vi "niRFUtil MT UTIL Calcuate PN Bits Galois.vi"(4 "primitive polynomial coeffs (without MSB)":u32, 6 "Reset? (T)":bool=TRUE, 9 "seed in (0xD6BF7DF2)":T4=3602873842 format="%.0x", 10 "PN Sequence Order (9)":T2=9, 11 "Total Bits":i32) -> (1 "seed out":T4 format="%.0x", 3 "Output Bit Stream":T3 min=0)   [LabVIEW 2015, in "niRFUtil.lvlib"]
doc: "This VI generates a pseudo-random bit stream. The length of the random sequence (i.e., the number of bits that are produced before the pattern repeats itself) is user-defined."
uses:
  niRFUtil.lvlib
  Includes/niRFUtil INC PN Seed.ctl
  Includes/niRFUtil INC Bit Array.ctl
  Includes/niRFUtil INC PN Order.ctl
panel:
  in  "Case Constant\n(See Context Help)":T1(ring)=enum."Shift Primative Seeds"
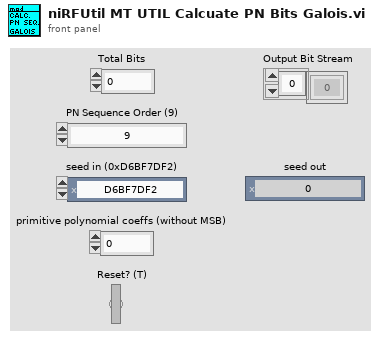
[diagram p1: front panel]
types:
  T1 = enum16{"Ver 2 Algorithm", "Shift Primative Seeds"}
  T2 = typedef "niRFUtil.lvlib/niRFUtil INC PN Order.ctl" = i32
  T3 = typedef "niRFUtil.lvlib/niRFUtil INC Bit Array.ctl" = i8[]
  T4 = typedef "niRFUtil.lvlib/niRFUtil INC PN Seed.ctl" = u32
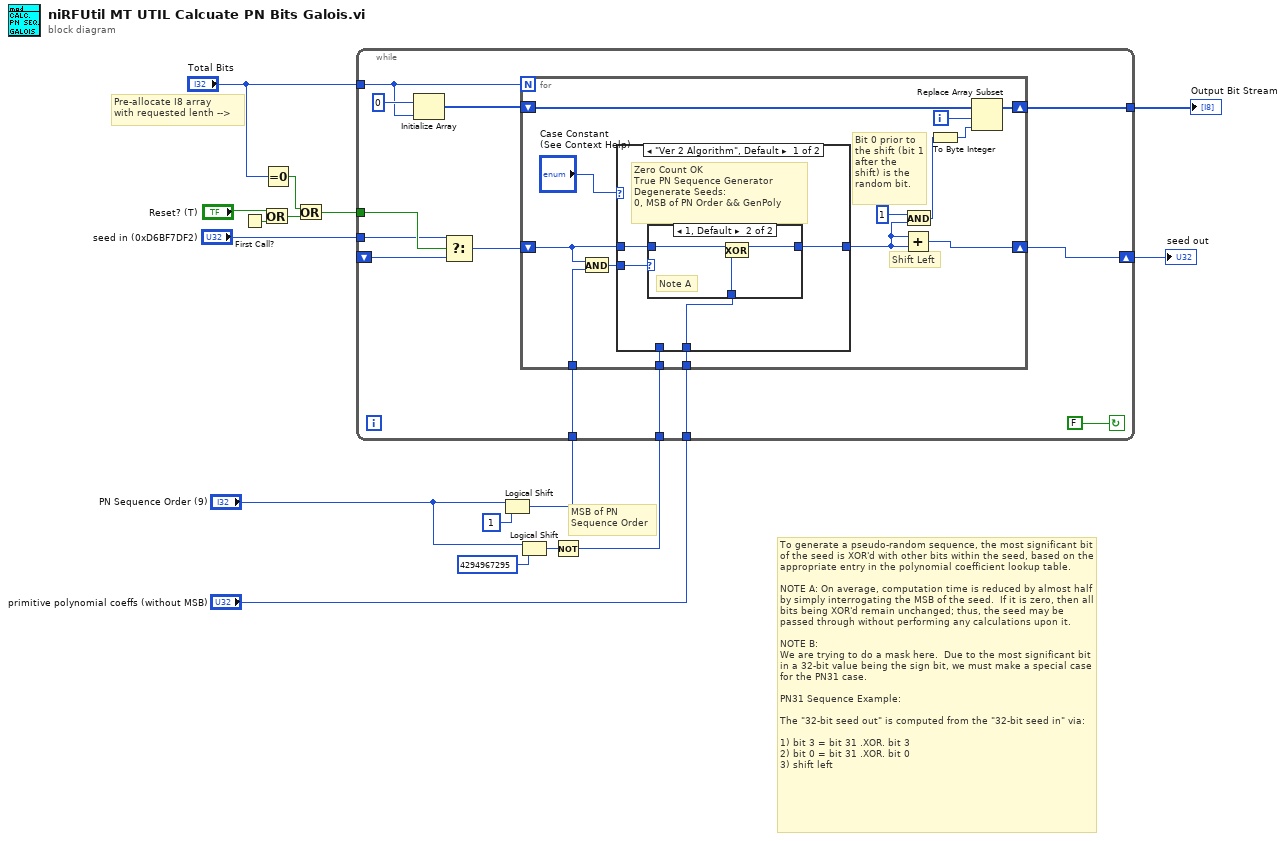
[diagram p0: block diagram]
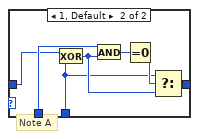
[diagram p4: hidden frame]
diagram:
  # "Pre-allocate I8 array \nwith requested lenth -->"
  # "MSB of PN\nSequence Order"
  # "To generate a pseudo-random sequence, the most significant bit of the seed is XOR'd with other bits within the seed, based on the appropriate entry in the polynomial coefficient lookup table.\n\nNOTE A: On average, computation time is reduced by almost half by simply interrogating the MSB of the seed.  If it is zero, then all bits being XOR'd remain unchanged; thus, the seed may be passed through without performing any calculations upon it.\n\nNOTE B:\nWe are trying to do a mask here.  Due to the most significant bit in a 32-bit value being the sign bit, we must make a special case for the PN31 case.\n\nPN31 Sequence Example:\n\nThe \"32-bit seed out\" is computed from the \"32-bit seed in\" via:\n\n1) bit 3 = bit 31 .XOR. bit 3\n2) bit 0 = bit 31 .XOR. bit 0\n3) shift left"
  n1 = First Call?() -> (First Call?: T/F=w8:bool)
  n2 = Or(x="Reset? (T)", y=w8) -> (x .or. y?=w5:bool)
  n3 = Equal To 0?(x="Total Bits") -> (x = 0?=w7:bool)
  n4 = Or(x=w7, y=w5) -> (x .or. y?=w4:bool)
  n5 = Logical Shift(y="PN Sequence Order (9)", x=u32 1) -> (x << y=w15:u32)
  n6 = Logical Shift(y="PN Sequence Order (9)", x=u32 4294967295) -> (x << y=w12:u32)
  n7 = Not(x=w12) -> (.not. x?=w11:u32)
  n8 = while {
    tunnel: w15 -> [w29]
    tunnel: w4 -> [w20]
    tunnel: [w26] -> w14
    tunnel: w11 -> [w25]
    tunnel: "primitive polynomial coeffs (without MSB)" -> [w24]
    tunnel: "Total Bits" -> [w23]
    shift-right: [w22] -> w1
    shift-left: _ -> [w18]
    tunnel: "seed in (0xD6BF7DF2)" -> [w19]
    stop <- FALSE continue-if-true
    n9 = Initialize Array(i8 0, w23) -> (w27:i8[])
    n10 = Select(t=w19, s=w20, f=w18) -> (s? t:f=w17:T4)
    n11 = for {
      N: w23 -> [_]
      shift-right: [w43] -> w22
      shift-left: w17 -> [w30]
      tunnel: w29 -> [w36]
      tunnel: w24 -> [w34]
      shift-right: [w39] -> w26
      shift-left: w27 -> [w40]
      tunnel: w25 -> [w37]
      i -> [w41]
      # "Shift Left"
      # "Bit 0 prior to the shift (bit 1 after the shift) is the random bit."
      n12 = And(x=w30, y=w36) -> (x .and. y?=w35:T4)
      n13 = case shown="\"Ver 2 Algorithm\", Default" "Case Constant\n(See Context Help)" {
        tunnel: [w45 w56] -> w31
        tunnel: w30 -> [w46 w55]
        tunnel: w37 -> [_ w54]
        tunnel: w35 -> [w47 w53]
        tunnel: w34 -> [w44 w52]
        frame "Ver 2 Algorithm", Default {
          # "Zero Count OK\nTrue PN Sequence Generator\nDegenerate Seeds: \n0, MSB of PN Order && GenPoly"
          n14 = case shown="1, Default" w47 {
            tunnel: [w48 w50] -> w45
            tunnel: w46 -> [w48 w51]
            tunnel: w44 -> [_ w49]
            frame 0 {
            }
            frame 1, Default {
              # "Note A"
              n15 = Exclusive Or(1:w49, 2:w51) -> (0:w50:T4)
            }
          }
        }
        frame "Shift Primative Seeds" {
          # "Revised Algorithm shifts the seed\nwhen input seed = GP"
          n16 = case shown="0" w53 {
            tunnel: [w57 w61] -> w56
            tunnel: w55 -> [w57 w60]
            tunnel: w52 -> [_ w58]
            tunnel: w54 -> [_ w64]
            frame 0 {
            }
            frame 1, Default {
              # "Note A"
              n17 = Exclusive Or(1:w58, 2:w60) -> (0:w59:T4)
              n18 = And(x=w64, y=w59) -> (x .and. y?=w63:T4)
              n19 = Equal To 0?(x=w63) -> (x = 0?=w62:bool)
              n20 = Select(t=w58, s=w62, f=w59) -> (s? t:f=w61:T4)
            }
          }
        }
      }
      n21 = Add(x=w31, y=w31) -> (x+y=w43:T4)
      n22 = And(x=u32 1 ("y"), y=w31) -> (x .and. y?=w42:T4)
      n23 = To Byte Integer(number=w42) -> (8bit integer=w38:i8)
      n24 = Replace Array Subset(array=w40, new element=w38, index=w41) -> (w39:i8[])
    }
  }
  "seed out" <- w1
  "Output Bit Stream" <- w14
